vi "RSC_Set_Parameters.vi"(8 "error in (no error)":errorcluster, 10 "Data to update":T1, 11 "Reward_SubCondition in":refnum<class "Reward_SubCondition.lvclass">) -> (0 "error out":errorcluster, 3 "Reward_SubCondition out":refnum<class "Reward_SubCondition.lvclass">)   [LabVIEW 2018, in "Tracker.lvlib" / "Reward_SubCondition.lvclass"]
uses:
  Reward_SubCondition.lvclass
  Reward_SubCondition.lvclass/Reward_SubCondition.ctl
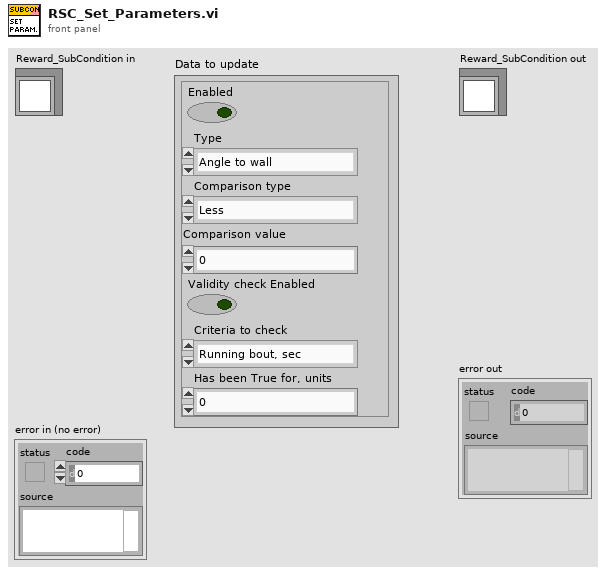
[diagram p1: front panel]
types:
  T1 = cluster{"Enabled":bool, "Type":enum16{"Angle to wall", "Speed", "Zone"}, "Comparison type":enum16{"Less", "Less or Equal", "Equal", "Greater or Equal", "Greater", "Not Equal"}, "Comparison value":dbl, "Validity check Enabled":bool, "Criteria to check":enum16{"Running bout, sec", "Running bout, m"}, "Has been True for, units":dbl}
  T2 = enum16{"Less", "Less or Equal", "Equal", "Greater or Equal", "Greater", "Not Equal"}
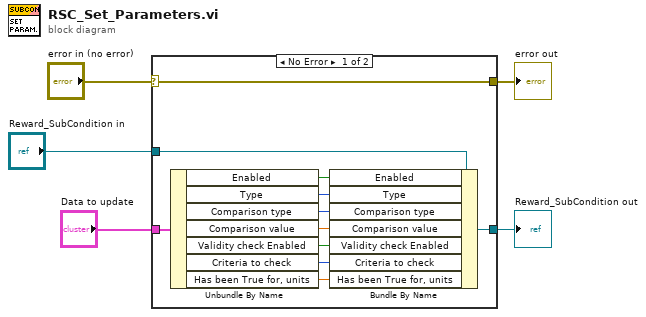
[diagram p0: block diagram]
diagram:
  n1 = case shown="No Error" "error in (no error)" {
    selector: "error in (no error)" -> [w16 w18]
    tunnel: [w16 w18] -> w4
    tunnel: [w14 w17] -> w2
    tunnel: "Reward_SubCondition in" -> [w15 w17]
    tunnel: "Data to update" -> [w13 _]
    frame No Error {
      n2 = Unbundle By Name(w13) -> ("Enabled"=w12:bool, "Type"=w11:enum16{"Angle to wall", "Speed", "Zone"}, "Comparison type"=w10:T2, "Comparison value"=w9:dbl, "Validity check Enabled"=w8:bool, "Criteria to check"=w7:enum16{"Running bout, sec", "Running bout, m"}, "Has been True for, units"=w6:dbl)
      n3 = Bundle By Name(cluster=w15, "Enabled"=w12, "Type"=w11, "Comparison type"=w10, "Comparison value"=w9, "Validity check Enabled"=w8, "Criteria to check"=w7, "Has been True for, units"=w6) -> (w14:refnum<class "Reward_SubCondition.lvclass">)
    }
    frame Error {
    }
  }
  "error out" <- w4
  "Reward_SubCondition out" <- w2
